vi "Controller Error Status BPM.vi"() -> ()   [LabVIEW 2011, in "Controller Global Variables.lvlib"]
uses:
  Controller Global Variables.lvlib
panel:
  in  "Controller Error Status BPM":u8[](array[numeric])
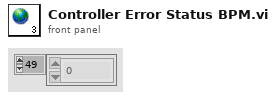
[diagram p1: front panel]
diagram:
